vi "doAction.vi"(8 "error in (no error)":errorcluster, 10 "ContextData":refnum<class "ContextData.lvclass">, 11 "User State 2 in":refnum<class "High Scores.lvclass">) -> (0 "error out":errorcluster, 2 "ContextData Out":refnum<class "ContextData.lvclass">, 3 "User State 2 out":refnum<class "High Scores.lvclass">)   [LabVIEW 2019, in "High Scores.lvclass"]
uses:
  High Scores.lvclass
  ContextData/ContextData.lvclass
  Player/Player.lvclass/Player.ctl
  Player/Player.lvclass
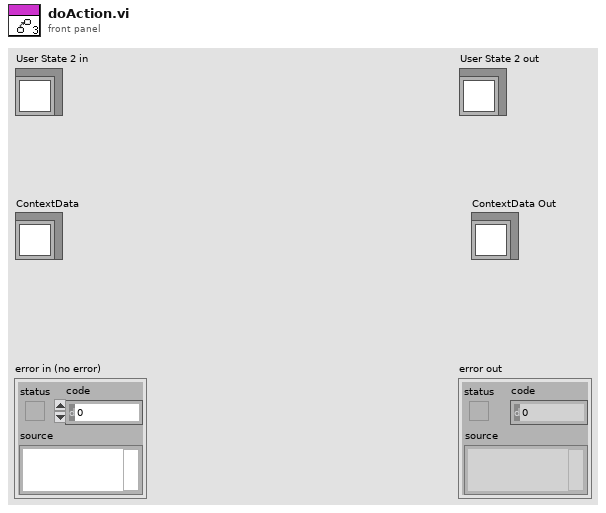
[diagram p1: front panel]
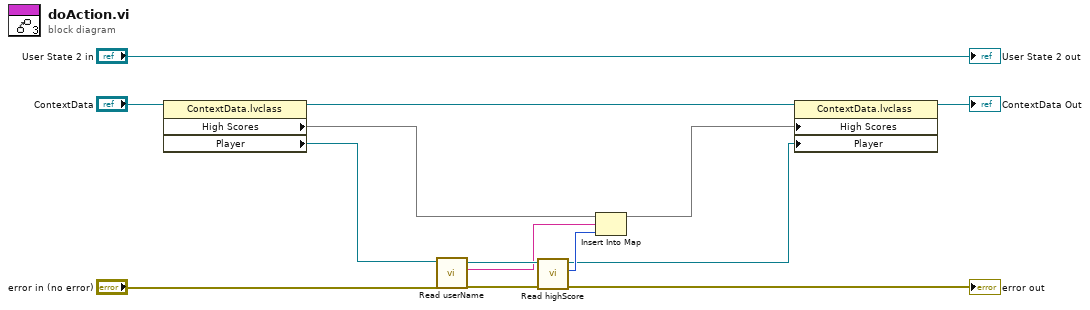
[diagram p0: block diagram]
diagram:
  n1 = property class="ContextData.lvclass"(reference="ContextData") -> (reference out=w12:refnum<class "ContextData.lvclass">, "High Scores"=w6:map{string, i32}, "Player"=w3:refnum<class "Player.lvclass">)  [unwired: 1 in, 1 out]
  n2 = call "Read userName.vi"("error in (no error)"="error in (no error)", "Player in"=w3) -> ("error out"=w9:errorcluster, "userName"=w8:string, "Player out"=w10:refnum<class "Player.lvclass">)  [unwired: 7 in]
  n3 = call "Read highScore.vi"("error in (no error)"=w9, "Player in"=w10) -> ("error out"=→"error out":errorcluster, "highScore"=w7:u64, "Player out"=w4:refnum<class "Player.lvclass">)  [unwired: 7 in]
  n4 = Insert Into Map(map in=w6, key=w8, value=w7) -> (map out=w5:map{string, i32})  [unwired: 2 out]
  n5 = property class="ContextData.lvclass"(reference=w12, "High Scores"=w5, "Player"=w4) -> (reference out=→"ContextData Out":refnum<class "ContextData.lvclass">)  [unwired: 1 in, 1 out]
  "User State 2 out" <- "User State 2 in"
